vi "Set Target Images.vi"() -> ()   [LabVIEW 2014]
uses:
  <vilib>/nisyscfg/Set System Image (File).vi
  <vilib>/nisyscfg/nisyscfg.lvlib
panel:
  in  "OK Button":bool
  in  "Session List":refnum<k21>[](array[refnum])
  in  "Source File":path caption="Image Location"
  # "Select Systems to Deploy Image to and then click OK"
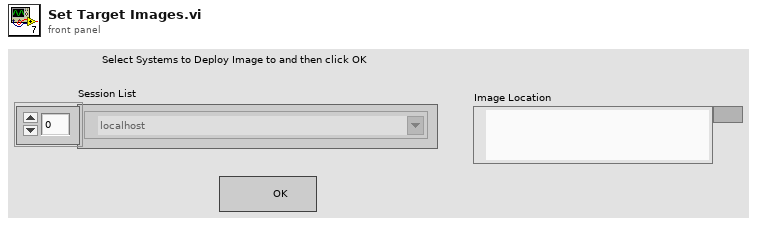
[diagram p1: front panel]
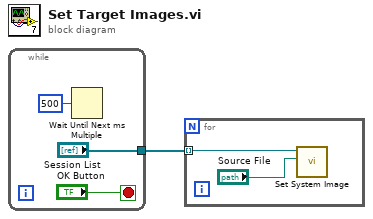
[diagram p0: block diagram]
diagram:
  n1 = while {
    tunnel: ["Session List"] -> w1
    stop <- "OK Button" stop-if-true
    n2 = Wait Until Next ms Multiple(millisecond multiple=u32 500) -> ()  [unwired: 1 out]
  }
  n3 = for {
    tunnel: w1 -> [w5] mode=indexing
    n4 = call-poly <vilib>:"Set System Image.vi"("Source File"="Source File", "Session in"=w5) -> ()  [unwired: 8 in, 2 out]
  }
